vi "_USB_CAN_DISP_ID_HB_.vi"(1 "Arr In":T1[](array[typedef])) -> (0 "Arr Out":T1[](array[typedef]))   [LabVIEW 2011]
uses:
  _USB_CAN_T_R_Unit_.ctl
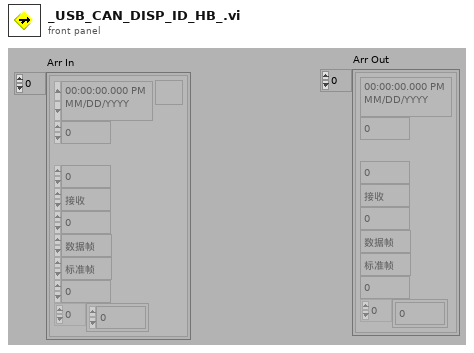
[diagram p1: front panel]
types:
  T1 = typedef "_USB_CAN_T_R_Unit_.ctl" = cluster{"time":timestamp, "channel":u16, "TimeStamp":u32, "tr":enum16{"接收", "发送"}, "id":u32, "Type":enum16{"数据帧", "远程帧"}, "Format":enum16{"标准帧", "扩展帧"}, "len":u8, "data":u8[]}
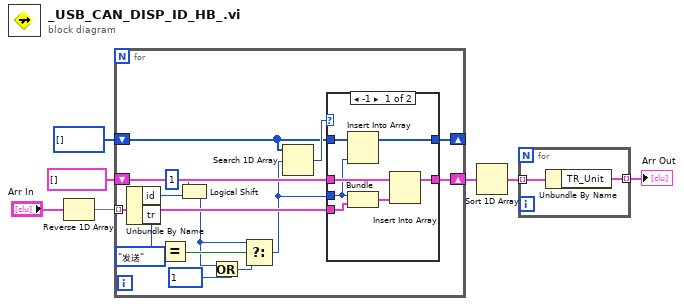
[diagram p0: block diagram]
diagram:
  n1 = Reverse 1D Array(array="Arr In") -> (reversed array=w5:T1[])
  n2 = for {
    tunnel: w5 -> [w17] mode=indexing
    shift-right: [w20] -> w4
    shift-left: cluster{"id":u32, "TR_Unit":T1}[] [] -> [w21]
    shift-right: [w18] -> _
    shift-left: u32[] [] -> [w19]
    n3 = Unbundle By Name(w17) -> ("id"=w12:u32, "tr"=w16:enum16{"接收", "发送"})
    n4 = Equal?(x=w16, y=enum16{"接收", "发送"}."发送") -> (x = y?=w14:bool)
    n5 = Logical Shift(y=i8 1, x=w12) -> (x << y=w9:u32)
    n6 = Or(x=w9, y=u32 1) -> (x .or. y?=w10:u32)
    n7 = Select(t=w9, s=w14, f=w10) -> (s? t:f=w13:u32)
    n8 = Search 1D Array(1D array=w19, element=w13) -> (index of element=w22:i32)  [unwired: 1 in]
    n9 = case shown="-1" w22 {
      tunnel: w13 -> [w25 _]
      tunnel: w21 -> [w27 w30]
      tunnel: [w26 w30] -> w20
      tunnel: w19 -> [w29 w31]
      tunnel: [w28 w31] -> w18
      tunnel: w17 -> [w24 _]
      frame -1 {
        n10 = Insert Into Array(array=w29, new element=w25) -> (w28:u32[])  [unwired: 1 in]
        n11 = Bundle(w25, "TR_Unit"=w24) -> (w23:cluster{u32, "TR_Unit":T1})  [unwired: 1 in]
        n12 = Insert Into Array(array=w27, new element=w23) -> (w26:cluster{"id":u32, "TR_Unit":T1}[])  [unwired: 1 in]
      }
      frame 0, Default {
      }
    }
  }
  n13 = Sort 1D Array(array=w4) -> (sorted array=w3:cluster{"id":u32, "TR_Unit":T1}[])
  n14 = for {
    tunnel: w3 -> [w33] mode=indexing
    tunnel: [w32] -> w2 mode=indexing
    n15 = Unbundle By Name(w33) -> ("TR_Unit"=w32:T1)
  }
  "Arr Out" <- w2
